vi "timeStampFromIMAQdx.vi"(7 "Image":T1, 8 "error in (no error)":errorcluster, 11 "IMAQdx Session":T2) -> (0 "error out":errorcluster, 1 "error occurred":bool, 3 "TimeStamp in Seconds":dbl, 4 "function execution time":u32)   [LabVIEW 2010]
uses:
  <vilib>/userDefined/High Color/IMAQdx.ctl
  <vilib>/vision/Image Controls.llb/IMAQ Image.ctl
  Program Files (x86)/National Instruments/LabVIEW 2010/resource/objmgr/imaqdx.rc
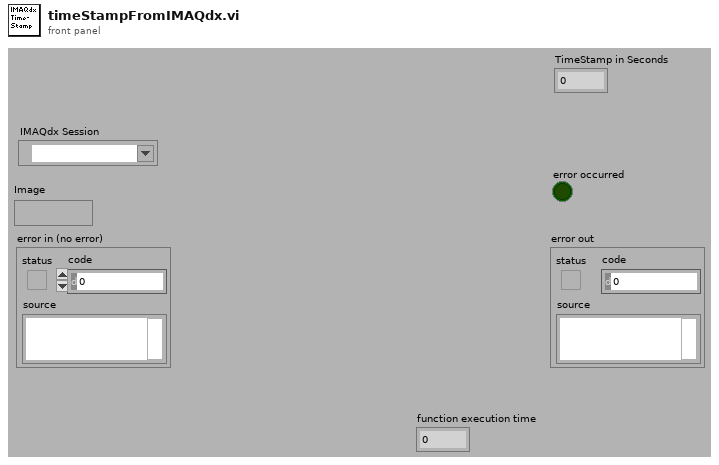
[diagram p1: front panel]
types:
  T1 = typedef "IMAQ Image.ctl" = refnum<image>
  T2 = typedef "IMAQdx.ctl" = refnum<k21>
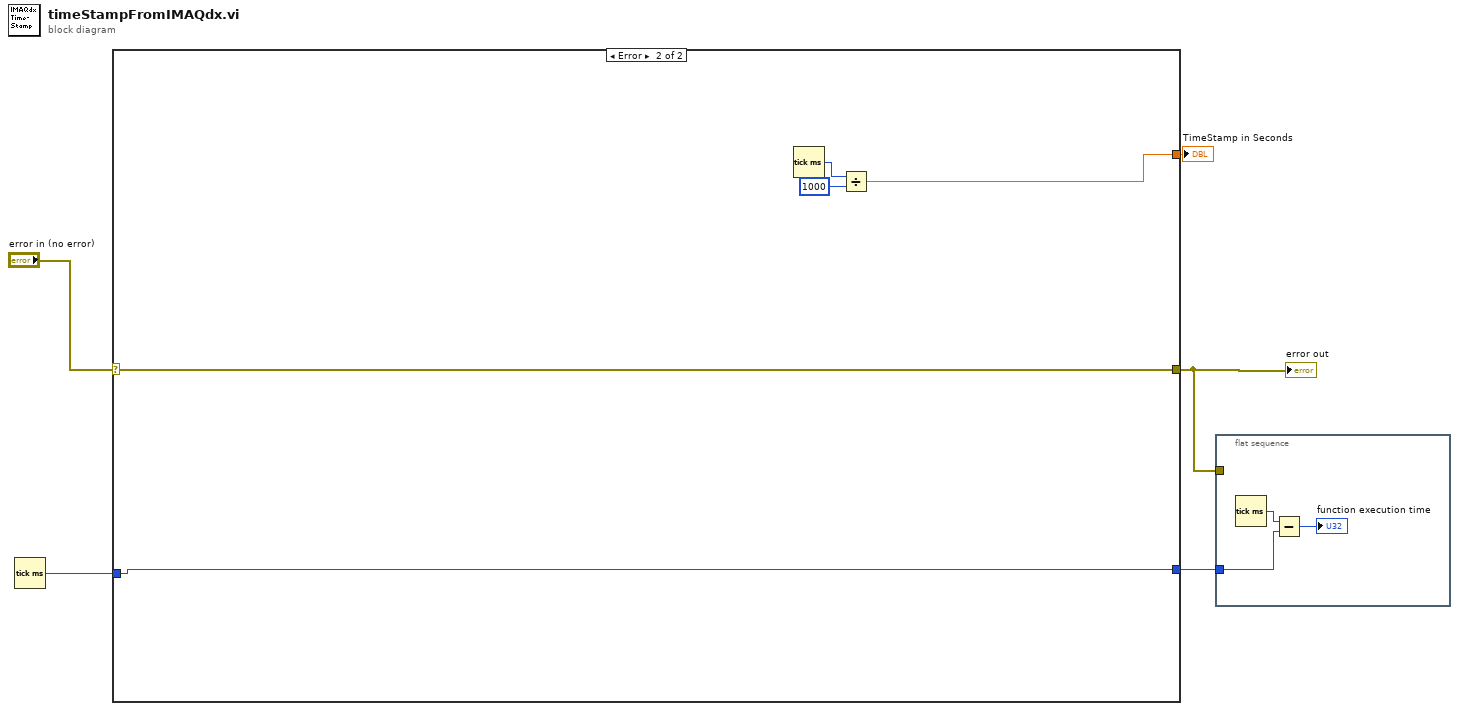
[diagram p0: block diagram]
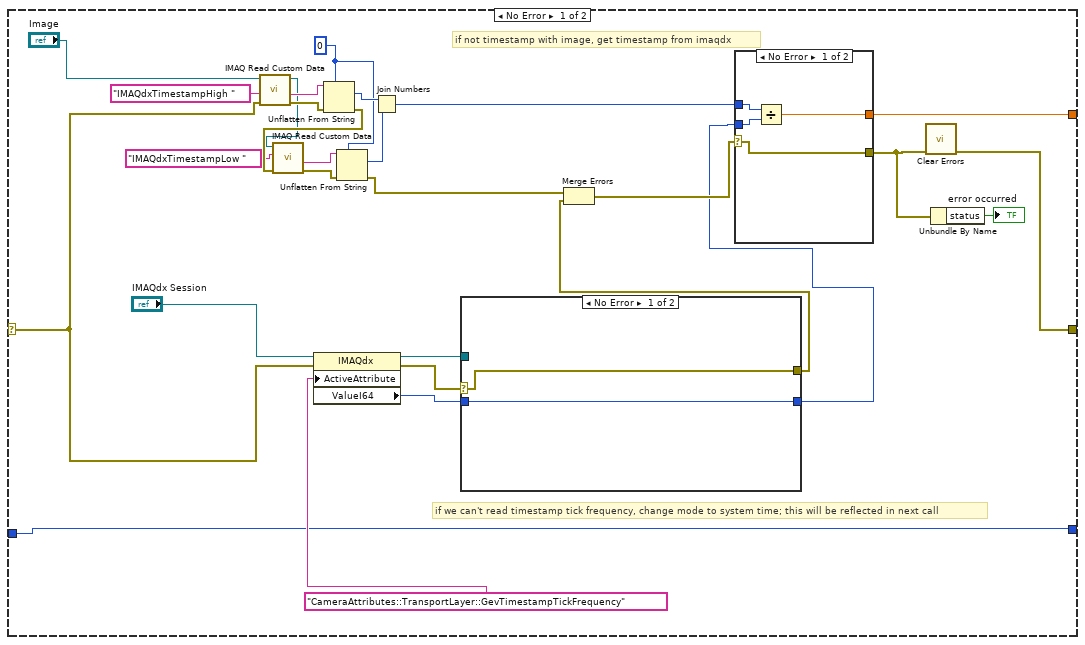
[diagram p2: hidden frame]
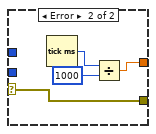
[diagram p3: hidden frame]
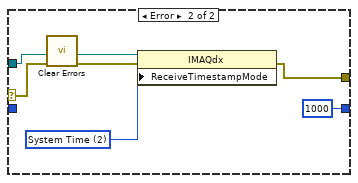
[diagram p4: hidden frame]
diagram:
  n1 = Tick Count (ms)() -> (millisecond timer value=w3:u32)
  n2 = case shown="Error" "error in (no error)" {
    selector: "error in (no error)" -> [w19 w51]
    tunnel: [w10 w52] -> w4
    tunnel: [w9 w51] -> w1
    tunnel: w3 -> [w6 w50]
    tunnel: [w6 w50] -> w2
    frame No Error {
      w24 = u32 0
      # "if not timestamp with image, get timestamp from imaqdx"
      # "if we can't read timestamp tick frequency, change mode to system time; this will be reflected in next call"
      n3 = call "IMAQ Read Custom Data"("error in (no error)"=w19, "Key"="IMAQdxTimestampHigh ", "Image"="Image") -> ("error out"=w30:errorcluster, "Custom Data Out"=w29:string, "Image (duplicate)"=w23:T1)  [unwired: 6 in]
      n4 = property class="IMAQdx"(reference="IMAQdx Session", error in=w19, "ActiveAttribute"="CameraAttributes::TransportLayer::GevTimestampTickFrequency") -> (reference out=w17:T2, error out=w16:errorcluster, "ValueI64"=w18:i64)
      n5 = Unflatten From String(type=w24, binary string=w29, error in (no error)=w30) -> (value=w28:u32, error out=w25:errorcluster)  [unwired: 2 in, 1 out]
      n6 = call "IMAQ Read Custom Data"("error in (no error)"=w25, "Key"="IMAQdxTimestampLow ", "Image"=w23) -> ("error out"=w27:errorcluster, "Custom Data Out"=w26:string)  [unwired: 6 in, 1 out]
      n7 = Unflatten From String(type=w24, binary string=w26, error in (no error)=w27) -> (value=w22:u32, error out=w15:errorcluster)  [unwired: 2 in, 1 out]
      n8 = Join Numbers(hi=w28, lo=w22) -> ((hi.lo)=w12:u64)
      n9 = case shown="No Error" w16 {
        selector: w16 -> [w42 w48]
        tunnel: w17 -> [_ w47]
        tunnel: w18 -> [w43 _]
        tunnel: [w42 w45] -> w14
        tunnel: [w43 i64 1000 ("ValueI64")] -> w11
        frame No Error {
        }
        frame Error {
          w49 = u32 2 items=["None", "Tick Count", "System Time"] ("ReceiveTimestampMode")
          n10 = call <vilib>:"Clear Errors.vi"("error in (no error)"=w48) -> ("error out"=w46:errorcluster)  [unwired: 6 in]
          n11 = property class="IMAQdx"(reference=w47, error in=w46, "ReceiveTimestampMode"=w49) -> (error out=w45:errorcluster)  [unwired: 1 out]
        }
      }
      n12 = Merge Errors(w15, w14) -> (w13:errorcluster)
      n13 = case shown="No Error" w13 {
        selector: w13 -> [w34 w38]
        tunnel: w12 -> [w36 _]
        tunnel: w11 -> [w37 _]
        tunnel: [w35 w39] -> w10
        tunnel: [w34 w38] -> w8
        frame No Error {
          n14 = Divide(x=w36, y=w37) -> (x/y=w35:dbl)
        }
        frame Error {
          n15 = Tick Count (ms)() -> (millisecond timer value=w41:u32)
          n16 = Divide(x=w41, y=u32 1000) -> (x/y=w39:dbl)
        }
      }
      n17 = call <vilib>:"Clear Errors.vi"("error in (no error)"=w8) -> ("error out"=w9:errorcluster)  [unwired: 6 in]
      n18 = Unbundle By Name(w8) -> ("status"=→"error occurred":bool)
    }
    frame Error {
      n19 = Tick Count (ms)() -> (millisecond timer value=w53:u32)
      n20 = Divide(x=w53, y=u32 1000) -> (x/y=w52:dbl)
    }
  }
  "TimeStamp in Seconds" <- w4
  "error out" <- w1
  n21 = flat-sequence {
    tunnel: w2 -> [w56]
    tunnel: w1 -> [_]
    frame #0 {
      n22 = Tick Count (ms)() -> (millisecond timer value=w57:u32)
      n23 = Subtract(x=w57, y=w56) -> (x-y=→"function execution time":u32)
    }
  }
